vi "getDeviceType.vi"(8 "error in (no error)":errorcluster, 11 "ethernetSupply.lvclass in":refnum<class "ethernetSupply.lvclass">) -> (0 "error out":errorcluster, 2 "type":T1(ring), 3 "ethernetSupply.lvclass out":refnum<class "ethernetSupply.lvclass">)   [LabVIEW 2011, in "Tools.lvlib" / "DatabaseHelpers.lvlib" / "ethernetSupply.lvclass"]
uses:
  ethernetSupply.lvclass
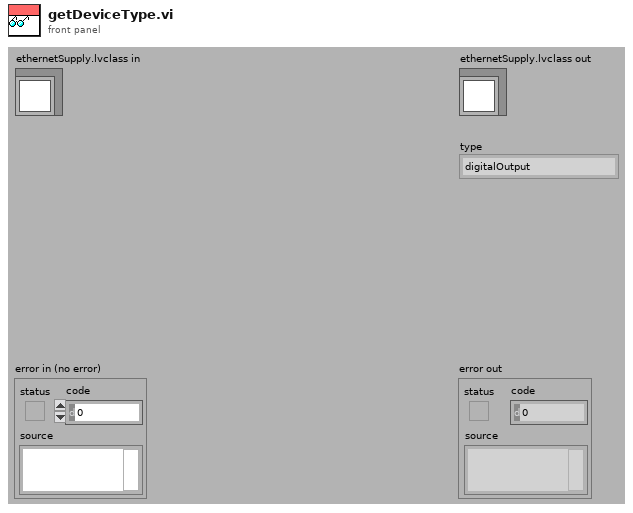
[diagram p1: front panel]
types:
  T1 = enum16{"digitalOutput", "digitalInput", "analogOutput", "analogInput", "rfOutput", "ethernetSupply"}
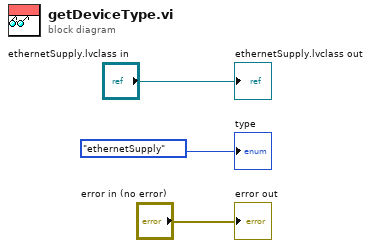
[diagram p0: block diagram]
diagram:
  "error out" <- "error in (no error)"
  "ethernetSupply.lvclass out" <- "ethernetSupply.lvclass in"
  "type" <- T1."ethernetSupply" ("type")
